vi "Verify Combinations.vi"(5 "Options":T1, 7 "Test VI (caller)":string, 8 "error in":errorcluster, 9 "map (control name -> array of variants)":map{string, variant[]}(c390), 10 "VI Refnum":refnum<vi>) -> (0 "error out":errorcluster)   [LabVIEW 2020, in "Caraya.Extension.lvlib"]
uses:
  Caraya.Extension.lvlib
  <vilib>/addons/_JKI Toolkits/Caraya/classes/Assert/Assert.lvclass
  <vilib>/addons/_JKI Toolkits/Caraya/classes/Assert/Assert True.vi
  Approval Tests/Approval Tests.lvlib
  Approval Tests/Reporter/Reporter.lvclass
  Approval Tests/Printer/Printer.lvclass
  Approval Tests/Options.ctl
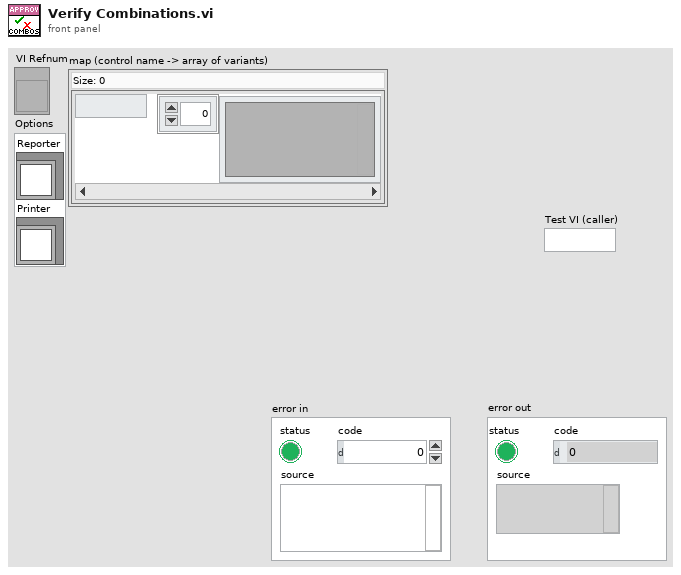
[diagram p1: front panel]
types:
  T1 = typedef "Approval Tests.lvlib/Options.ctl" = cluster{"Reporter":refnum<class "Reporter.lvclass">, "Printer":refnum<class "Printer.lvclass">}
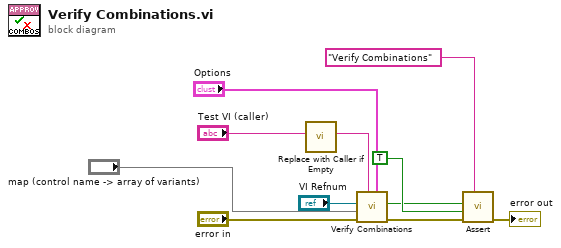
[diagram p0: block diagram]
diagram:
  n1 = call "Replace with Caller if Empty.vi"("Test VI (caller) in"="Test VI (caller)") -> ("Test VI (caller) out"=w4:string)  [unwired: 10 in]
  n2 = call "Verify Combinations.vi"("Options"="Options", "Test VI (caller)"=w4, "error in (no error)"="error in", "map (control name -> array of variants)"="map (control name -> array of variants)", "VI Refnum"="VI Refnum") -> ("error out"=w1:errorcluster, "Passed?"=w2:bool)  [unwired: 4 in, 1 out]
  n3 = call-poly <vilib>:"Assert.vi"("Label"="Verify Combinations", "error in (no error)"=w1, "Register with caller test (F)"=TRUE, "True?"=w2) -> ("error out"=→"error out":errorcluster)  [unwired: 6 in, 1 out]
